vi "HEWH Tank Display by Ref.vi"(5 "T1-T6.Tin,Tout":dbl[](array[numeric]), 6 "Tank Display":T1 {"TIN" format="%.2g"; "TOUT" format="%.2g"; "Mean" format="%.2f"; "Std Dev" format="%.2f"; "TC6" format="%.2g"; "TC5" format="%.2g"; "TC4" format="%.2g"; "TC3" format="%.2g"; "TC2" format="%.2g"; "TC1" format="%.2g"}, 7 "Min Temp (°F)":dbl=50.0, 9 "Max Temp (°F)":dbl=140.0, 11 "error in":errorcluster) -> (15 "error out":errorcluster)   [LabVIEW 2009]
uses:
  <vilib>/Analysis/NI_AALBase.lvlib
  HEWH Tank Indicator.ctl
panel:
  in  "Tank Display 2":refnum<vi>
  in  "Ctrl Reference":refnum<vi>
  out "Array 2":string[](array[string])
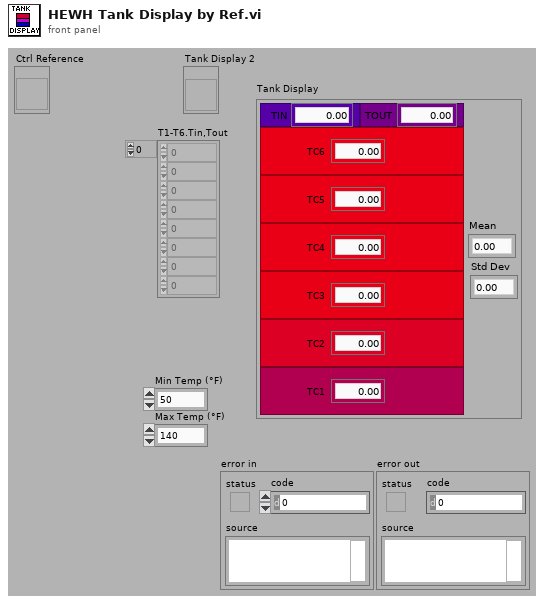
[diagram p1: front panel]
types:
  T1 = typedef "HEWH Tank Indicator.ctl" = cluster{"TC1-D":bool, "TC2-D":bool, "TC3-D":bool, "TC4-D":bool, "TC5-D":bool, "TC6-D":bool, "RTD_IN":bool, "RTDOUT":bool, "TC1":dbl, "TC2":dbl, "TC3":dbl, "TC4":dbl, "TC5":dbl, "TC6":dbl, "TIN":dbl, "TOUT":dbl, "Std Dev":dbl, "Mean":dbl}
  T2 = cluster{"T1-T6.Tin,Tout[0]":dbl, "T1-T6.Tin,Tout[1]":dbl, "T1-T6.Tin,Tout[2]":dbl, "T1-T6.Tin,Tout[3]":dbl, "T1-T6.Tin,Tout[4]":dbl, "T1-T6.Tin,Tout[5]":dbl, "T1-T6.Tin,Tout[6]":dbl, "T1-T6.Tin,Tout[7]":dbl}
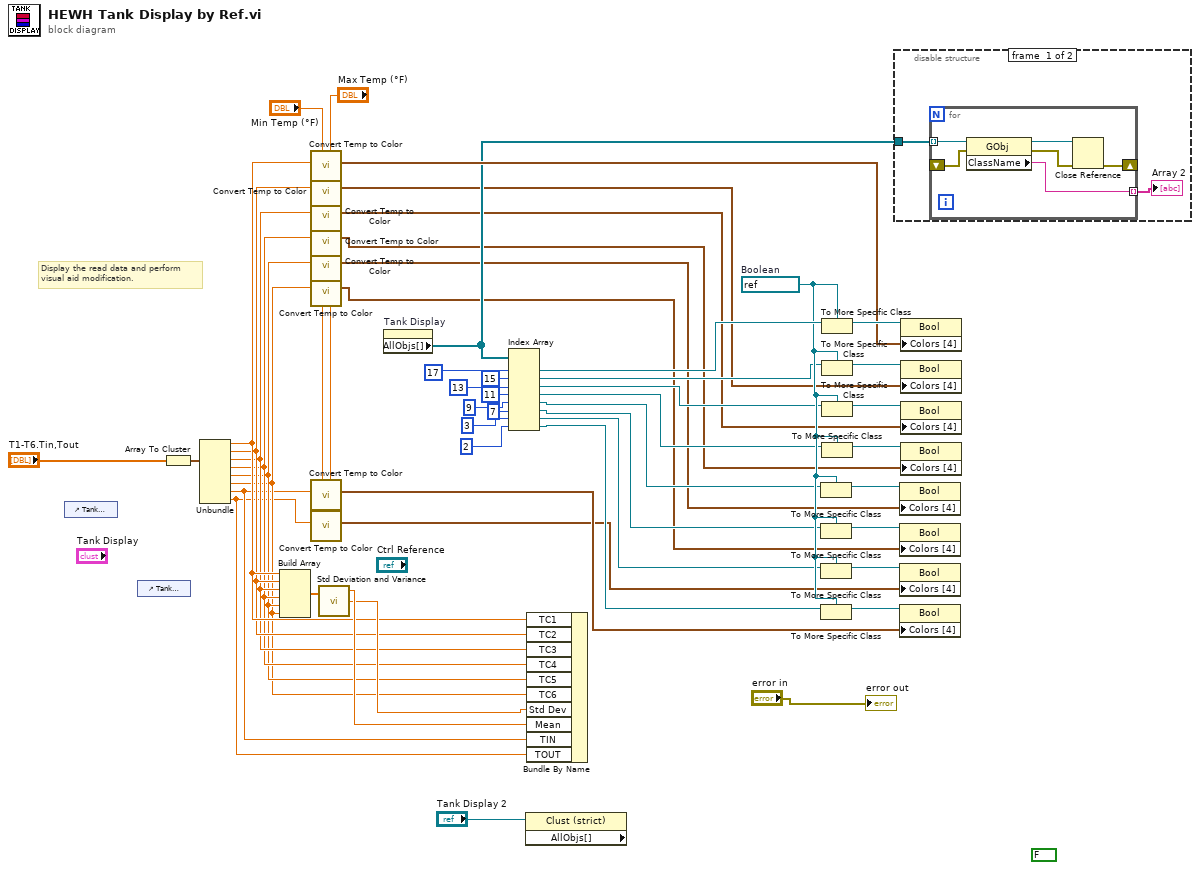
[diagram p0: block diagram]
diagram:
  w28 = refnum<vi> refnum  # Boolean
  (unwired) FALSE
  # "Display the read data and perform\nvisual aid modification."
  n1 = control-ref of="Tank Display"() -> (w2:refnum<vi>)
  n2 = control-ref of="Tank Display"() -> ()  [unwired: 1 out]
  n3 = Array To Cluster(array="T1-T6.Tin,Tout") -> (cluster=w56:T2)
  n4 = Unbundle(w56) -> ("T1-T6.Tin,Tout[0]"=w41:dbl, "T1-T6.Tin,Tout[1]"=w40:dbl, "T1-T6.Tin,Tout[2]"=w39:dbl, "T1-T6.Tin,Tout[3]"=w38:dbl, "T1-T6.Tin,Tout[4]"=w37:dbl, "T1-T6.Tin,Tout[5]"=w36:dbl, "T1-T6.Tin,Tout[6]"=w8:dbl, "T1-T6.Tin,Tout[7]"=w7:dbl)
  n5 = Build Array(w41, w40, w39, w38, w37, w36) -> (w67:dbl[])
  n6 = call "Convert Temp to Color.vi"("Max Temp (°F)"="Max Temp (°F)", "Min Temp (°F)"="Min Temp (°F)", "Temp (°F)"=w41) -> ("Color Output"=w50:cluster{"Color":u32, "Color":u32}[], "Max Temp (°F) Out"=w58:dbl, "Min Temp (°F) Out"=w57:dbl)  [unwired: 6 out]
  n7 = call "Convert Temp to Color.vi"("Max Temp (°F)"=w58, "Min Temp (°F)"=w57, "Temp (°F)"=w40) -> ("Color Output"=w20:cluster{"Color":u32, "Color":u32}[], "Max Temp (°F) Out"=w60:dbl, "Min Temp (°F) Out"=w59:dbl)  [unwired: 6 out]
  n8 = call "Convert Temp to Color.vi"("Max Temp (°F)"=w60, "Min Temp (°F)"=w59, "Temp (°F)"=w39) -> ("Color Output"=w19:cluster{"Color":u32, "Color":u32}[], "Max Temp (°F) Out"=w62:dbl, "Min Temp (°F) Out"=w61:dbl)  [unwired: 6 out]
  n9 = call "Convert Temp to Color.vi"("Max Temp (°F)"=w62, "Min Temp (°F)"=w61, "Temp (°F)"=w38) -> ("Color Output"=w18:cluster{"Color":u32, "Color":u32}[], "Max Temp (°F) Out"=w64:dbl, "Min Temp (°F) Out"=w63:dbl)  [unwired: 6 out]
  n10 = call "Convert Temp to Color.vi"("Max Temp (°F)"=w64, "Min Temp (°F)"=w63, "Temp (°F)"=w37) -> ("Color Output"=w17:cluster{"Color":u32, "Color":u32}[], "Max Temp (°F) Out"=w66:dbl, "Min Temp (°F) Out"=w65:dbl)  [unwired: 6 out]
  n11 = call "Convert Temp to Color.vi"("Max Temp (°F)"=w66, "Min Temp (°F)"=w65, "Temp (°F)"=w36) -> ("Color Output"=w16:cluster{"Color":u32, "Color":u32}[], "Max Temp (°F) Out"=w14:dbl, "Min Temp (°F) Out"=w15:dbl)  [unwired: 6 out]
  n12 = call "Convert Temp to Color.vi"("Max Temp (°F)"=w14, "Min Temp (°F)"=w15, "Temp (°F)"=w8) -> ("Color Output"=w6:cluster{"Color":u32, "Color":u32}[], "Max Temp (°F) Out"=w12:dbl, "Min Temp (°F) Out"=w13:dbl)  [unwired: 6 out]
  n13 = call "Convert Temp to Color.vi"("Max Temp (°F)"=w12, "Min Temp (°F)"=w13, "Temp (°F)"=w7) -> ("Color Output"=w5:cluster{"Color":u32, "Color":u32}[])  [unwired: 8 out]
  n14 = call <vilib>:"Std Deviation and Variance.vi"("X"=w67) -> ("mean"=w55:dbl, "standard deviation"=w54:dbl)  [unwired: 1 in, 1 out]
  n15 = property on="Tank Display" class="Clust (strict)"() -> ("AllObjs[]"=w49:refnum<vi>[])  [unwired: 2 in, 2 out]
  n16 = Index Array(array=w49, index #1=17 ("index"), index #2=15 ("index"), index #3=13 ("index"), index #4=11 ("index"), index #5=9 ("index"), index #6=7 ("index"), index #7=3 ("index"), index #8=2 ("index")) -> (element #1=w52:refnum<vi>, element #2=w27:refnum<vi>, element #3=w26:refnum<vi>, element #4=w25:refnum<vi>, element #5=w24:refnum<vi>, element #6=w23:refnum<vi>, element #7=w22:refnum<vi>, element #8=w21:refnum<vi>)
  n17 = property class="Clust (strict)" props=["AllObjs[]"](reference="Tank Display 2") -> ()  [unwired: 1 in, 3 out]
  n18 = Bundle By Name("TC1"=w41, "TC2"=w40, "TC3"=w39, "TC4"=w38, "TC5"=w37, "TC6"=w36, "Std Dev"=w54, "Mean"=w55, "TIN"=w8, "TOUT"=w7) -> (w3:cluster{})  [unwired: 1 out]
  n19 = To More Specific Class(target class=w28, reference=w24) -> (specific class reference=w32:refnum<vi>)  [unwired: 1 in, 1 out]
  n20 = To More Specific Class(target class=w28, reference=w23) -> (specific class reference=w31:refnum<vi>)  [unwired: 1 in, 1 out]
  n21 = To More Specific Class(target class=w28, reference=w22) -> (specific class reference=w30:refnum<vi>)  [unwired: 1 in, 1 out]
  n22 = To More Specific Class(target class=w28, reference=w21) -> (specific class reference=w29:refnum<vi>)  [unwired: 1 in, 1 out]
  n23 = To More Specific Class(target class=w28, reference=w52) -> (specific class reference=w51:refnum<vi>)  [unwired: 1 in, 1 out]
  n24 = To More Specific Class(target class=w28, reference=w27) -> (specific class reference=w35:refnum<vi>)  [unwired: 1 in, 1 out]
  n25 = To More Specific Class(target class=w28, reference=w26) -> (specific class reference=w34:refnum<vi>)  [unwired: 1 in, 1 out]
  n26 = To More Specific Class(target class=w28, reference=w25) -> (specific class reference=w33:refnum<vi>)  [unwired: 1 in, 1 out]
  n27 = disable-structure shown="Enabled" {
    disable-tunnel: w49 -> [w68 _]
    frame #0 {
      n28 = for {
        tunnel: w68 -> [w72] mode=indexing
        shift-right: [w75] -> _
        shift-left: _ -> [w71]
        tunnel: [w74] -> w69 mode=indexing
        n29 = property on="Property Node" class="GObj"(reference=w72, error in=w71) -> (reference out=w70:refnum<vi>, error out=w73:errorcluster, "ClassName"=w74:string)
        n30 = Close Reference(reference=w70, error in (no error)=w73) -> (error out=w75:errorcluster)
      }
      "Array 2" <- w69
    }
    frame #1 {
      # "This is used to find bools in cluster.  Note\nbug in Labview doesnt show array cluster\nobjects in correct order."
    }
  }
  n31 = property on="Property Node" class="Bool"(reference=w32, "Colors [4]"=w17) -> ()  [unwired: 1 in, 2 out]
  n32 = property on="Property Node" class="Bool"(reference=w31, "Colors [4]"=w16) -> ()  [unwired: 1 in, 2 out]
  n33 = property on="Property Node" class="Bool"(reference=w30, "Colors [4]"=w5) -> ()  [unwired: 1 in, 2 out]
  n34 = property on="Property Node" class="Bool"(reference=w29, "Colors [4]"=w6) -> ()  [unwired: 1 in, 2 out]
  n35 = property on="Property Node" class="Bool"(reference=w51, "Colors [4]"=w50) -> ()  [unwired: 1 in, 2 out]
  n36 = property on="Property Node" class="Bool"(reference=w35, "Colors [4]"=w20) -> ()  [unwired: 1 in, 2 out]
  n37 = property on="Property Node" class="Bool"(reference=w34, "Colors [4]"=w19) -> ()  [unwired: 1 in, 2 out]
  n38 = property on="Property Node" class="Bool"(reference=w33, "Colors [4]"=w18) -> ()  [unwired: 1 in, 2 out]
  "error out" <- "error in"
